vi "Test Clone Registration API.vi"() -> ()   [LabVIEW 2025, in "USB IO.lvlib"]
doc: "Tester for the cloneable module registry VIs.\n_____\nBased on DQMH Dev Tools: Project Template 7.1.2.1547."
uses:
  USB IO.lvlib
  Clone Registration.lvlib
panel:
  out "ID (All)":i32[](array[numeric])
  out "First (All)":bool[](array[boolean])
  out "Empty?":bool
  out "First?":bool
  out "replaced?":bool
  in  "Remove Module":bool
  in  "Add Module":bool
  in  "Module ID":i32
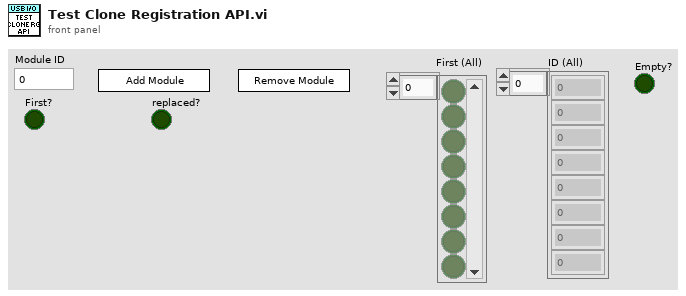
[diagram p1: front panel]
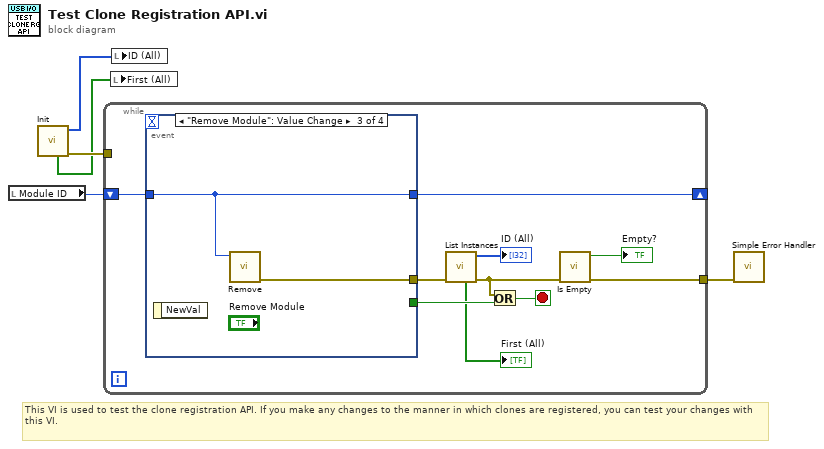
[diagram p0: block diagram]
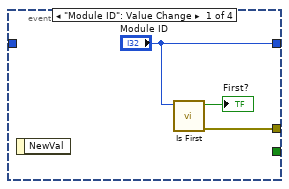
[diagram p2: hidden frame]
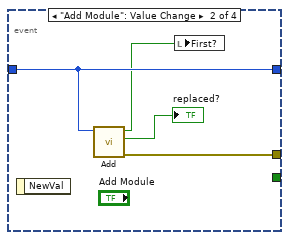
[diagram p3: hidden frame]
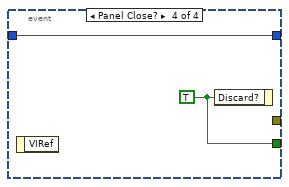
[diagram p4: hidden frame]
diagram:
  # "This VI is used to test the clone registration API. If you make any changes to the manner in which clones are registered, you can test your changes with this VI."
  n1 = local read "Module ID"() -> (w5:i32)
  n2 = call "Init.vi"() -> ("error out"=w3:errorcluster, "Module IDs"=w2:i32[], "First? (all)"=w1:bool[])  [unwired: 8 in, 1 out]
  n3 = while {
    shift-right: [w14] -> _
    shift-left: w5 -> [w13]
    tunnel: w3 -> [_]
    tunnel: [w9] -> w4
    stop <- w12 stop-if-true
    n4 = event shown="[2] \"Remove Module\": Value Change" {
      selector: _ -> [_ _ _ _]
      dyn-events: _ -> [_ _ _ _]
      timeout: _ -> [_ _ _ _]
      tunnel: [_ _ _ w26] -> w15
      tunnel: ["Module ID" w22 w23 w25] -> w14
      tunnel: w13 -> [_ w22 w23 w25]
      tunnel: [w16 w19 w24 _] -> w11
      event "Module ID": Value Change {
        n5 = event-data() -> ()  [unwired: 1 in, 1 out]
        n6 = call "Is First.vi"("Module ID"="Module ID") -> ("error out"=w16:errorcluster, "First?"=→"First?":bool)  [unwired: 9 in]
      }
      event "Add Module": Value Change {
        n7 = event-data() -> ()  [unwired: 1 in, 1 out]
        n8 = call "Add.vi"("Module ID"=w22) -> ("error out"=w19:errorcluster, "replaced?"=→"replaced?":bool, "First?"=w21:bool)  [unwired: 8 in]
        n9 = local write "First?"(w21) -> ()
      }
      event "Remove Module": Value Change {
        n10 = event-data() -> ()  [unwired: 1 in, 1 out]
        n11 = call "Remove.vi"("Module ID"=w23) -> ("error out"=w24:errorcluster)  [unwired: 9 in, 1 out]
      }
      event Panel Close? {
        w26 = TRUE ("Discard?")
        n12 = event-data() -> ()  [unwired: 1 in, 1 out]
        n13 = event-data("Discard?"=w26) -> ()  [unwired: 1 in, 1 out]
      }
    }
    n14 = call "List Instances.vi"("error in"=w11) -> ("error out"=w10:errorcluster, "Module IDs"=→"ID (All)":i32[], "First?"=→"First (All)":bool[])  [unwired: 6 in, 2 out]
    n15 = Or(x=w10, y=w15) -> (x .or. y?=w12:bool)
    n16 = call "Is Empty.vi"("error in"=w10) -> ("error out"=w9:errorcluster, "Empty?"=→"Empty?":bool)  [unwired: 9 in]
  }
  n17 = local write "First (All)"(w1) -> ()
  n18 = local write "ID (All)"(w2) -> ()
  n19 = call <vilib>:"Simple Error Handler.vi"("error in (no error)"=w4) -> ()  [unwired: 4 in, 5 out]
